vi "Configure Modulation (Amplitude).vi"(0 "VISA resource name":refnum<visa-resource-name>, 1 "Enable AM (T:Enable)":bool=TRUE, 2 "AM Path (1)":u16(ring)=1 items=["1"=1, "2"=2, "Wideband"=3], 5 "AM Mode (1: Normal)":u16(ring)=1 items=["Deep", "Normal"], 7 "AM Type (0: Linear)":u16(ring) items=["Linear", "Exponential"], 9 "Enable Depth Coupling (T:Enable)":bool=TRUE, 11 "error in (no error)":errorcluster, 12 "AM Depth (10 percent)":dbl=10.0, 13 "Wideband AM Sensitivity (20 dB)":dbl=20.0) -> (4 "VISA resource name out":refnum<visa-resource-name>, 15 "error out":errorcluster)   [LabVIEW 2018, in "Agilent PSG MXG Series.lvlib"]
doc: "Configures amplitude modulation.\n\n<B>Notes:</B>\n(1) This VI is <B>NOT</B> valid in E8247C.\n\n(2) For E8257D, E8267D, N5161A, N5162A, N5181A, N5182A, N5183A, this VI is valid only when the instument installs <B>Option UNT</B> (AM, FM, phase modulation).\n\n(3) For N5171B, N5172B, N5181B, N5182B, N5173B, N5183B, this VI is valid only when the instument installs <B>Option UNT</B> (AM, FM, phase modulation)."
uses:
  Agilent PSG MXG Series.lvlib
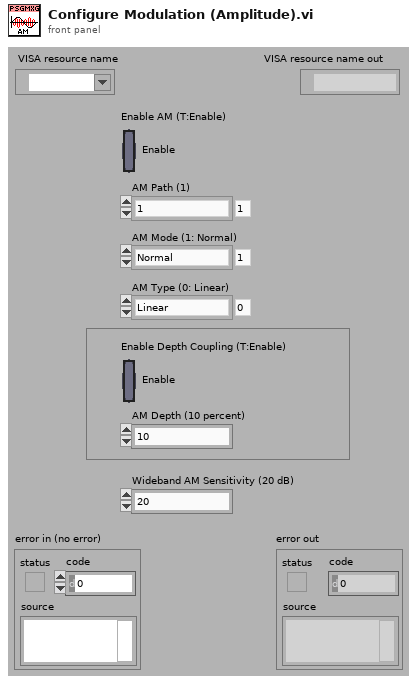
[diagram p1: front panel]
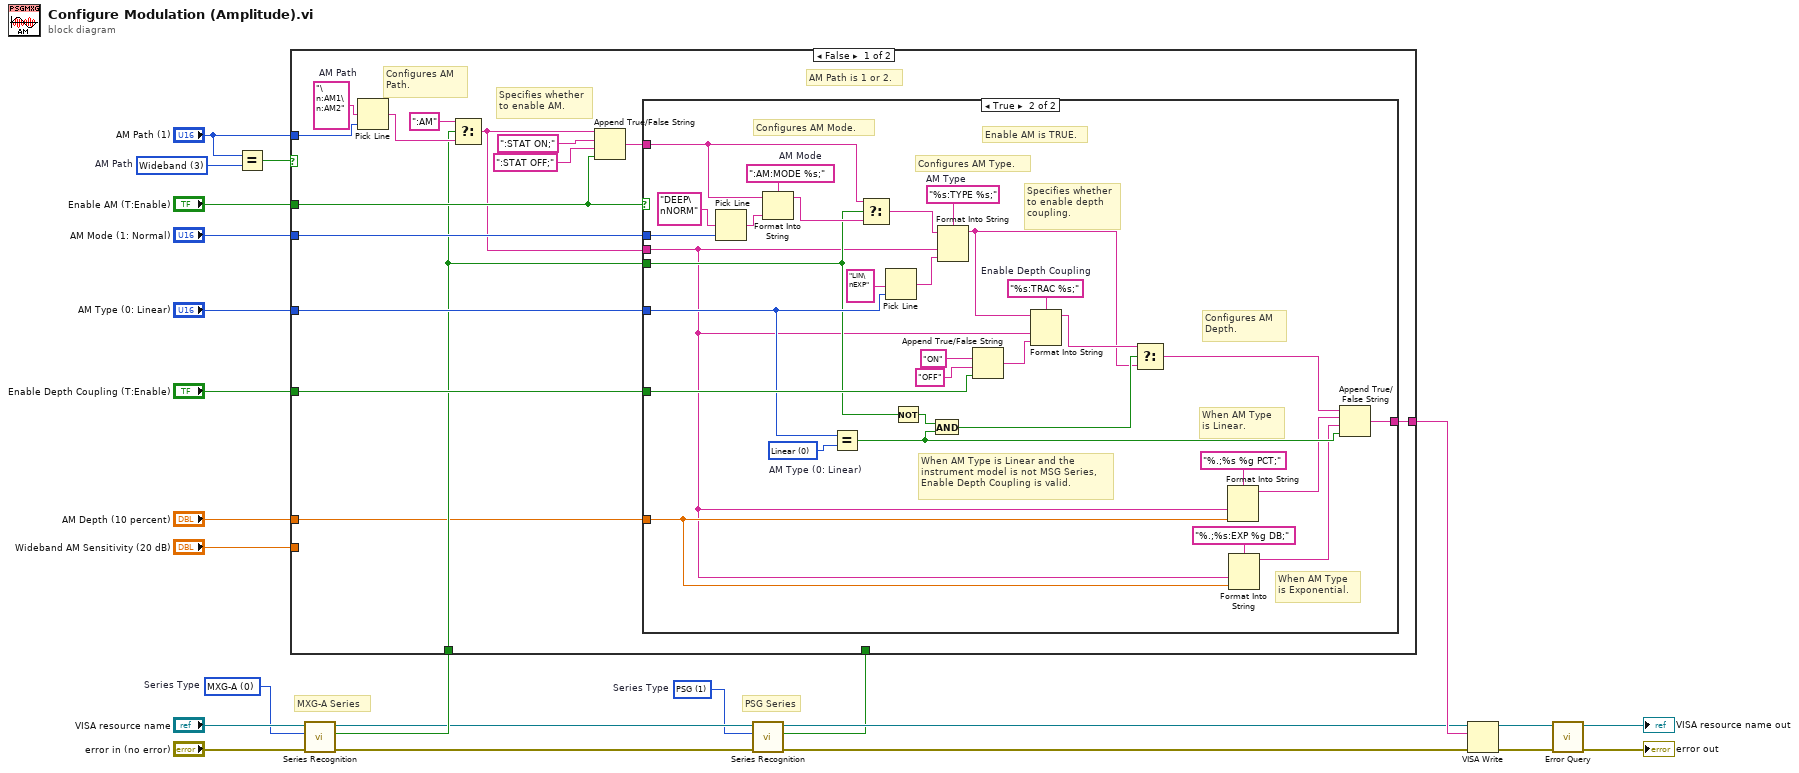
[diagram p0: block diagram]
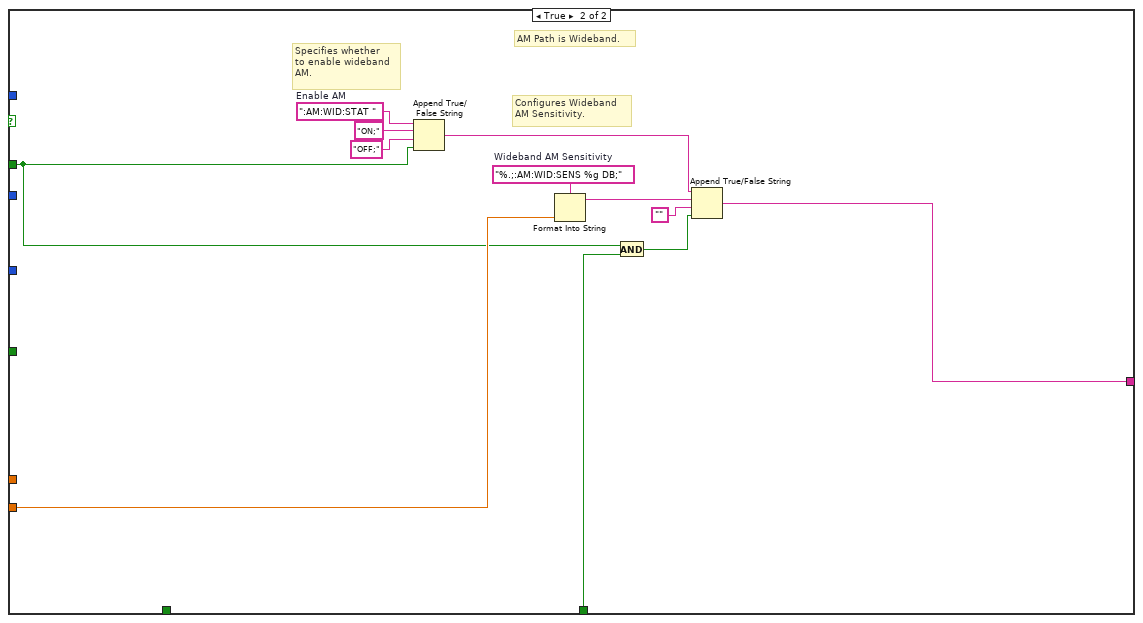
[diagram p3: hidden frame]
diagram:
  w5 = u16 1 items=["MXG-A", "PSG", "PSG-A", "PSG-C", "PSG-D", "MXG-B", "EXG"]  # Series Type
  w8 = u16 0 items=["MXG-A", "PSG", "PSG-A", "PSG-C", "PSG-D", "MXG-B", "EXG"]  # Series Type
  w24 = u16 3 items=["1"=1, "2"=2, "Wideband"=3]  # AM Path
  # "PSG Series"
  # "MXG-A Series"
  n1 = Equal?(x="AM Path (1)", y=w24) -> (x = y?=w23:bool)
  n2 = call "Series Recognition.vi"("error in (no error)"="error in (no error)", "Series Type (0: MXG)"=w8, "VISA resource name"="VISA resource name") -> ("error out"=w6:errorcluster, "Is Series Correct"=w13:bool, "VISA resource name out"=w7:refnum<visa-resource-name>)  [unwired: 6 out]
  n3 = call "Series Recognition.vi"("error in (no error)"=w6, "Series Type (0: MXG)"=w5, "VISA resource name"=w7) -> ("error out"=w2:errorcluster, "Is Series Correct"=w1:bool, "VISA resource name out"=w3:refnum<visa-resource-name>)  [unwired: 6 out]
  n4 = case shown="False" w23 {
    tunnel: "AM Path (1)" -> [w38 _]
    tunnel: "Enable AM (T:Enable)" -> [w32 w76]
    tunnel: "AM Mode (1: Normal)" -> [w35 _]
    tunnel: w13 -> [w29 _]
    tunnel: "AM Type (0: Linear)" -> [w31 _]
    tunnel: "Enable Depth Coupling (T:Enable)" -> [w30 _]
    tunnel: "AM Depth (10 percent)" -> [w27 _]
    tunnel: [w26 w72] -> w4
    tunnel: "Wideband AM Sensitivity (20 dB)" -> [_ w79]
    tunnel: w1 -> [_ w77]
    frame False {
      w39 = "\n:AM1\n:AM2"  # AM Path
      # "Specifies whether\nto enable AM."
      # "Configures AM\nPath."
      # "AM Path is 1 or 2."
      n5 = Pick Line(multi-line string=w39, line index=w38) -> (output string=w34:string)  [unwired: 1 out]
      n6 = Select(t=":AM", s=w29, f=w34) -> (s? t:f=w28:string)
      n7 = Append True/False String(1:w32, 2:":STAT OFF;" ("false string"), 3:":STAT ON;" ("true string"), 4:w28) -> (0:w36:string)
      n8 = case shown="True" w32 {
        tunnel: w36 -> [w40 w67]
        tunnel: w35 -> [_ w68]
        tunnel: w29 -> [_ w53]
        tunnel: w31 -> [_ w56]
        tunnel: w28 -> [_ w41]
        tunnel: w30 -> [_ w57]
        tunnel: w27 -> [_ w47]
        tunnel: [w40 w42] -> w26
        frame False {
          # "Enable AM is FALSE."
        }
        frame True {
          w55 = u16 0 items=["Linear", "Exponential"]  # AM Type (0: Linear)
          w61 = "%s:TRAC %s;"  # Enable Depth Coupling
          w64 = "%s:TYPE %s;"  # AM Type
          w71 = ":AM:MODE %s;"  # AM Mode
          # "When AM Type\nis Exponential."
          # "When AM Type\nis Linear."
          # "Configures AM\nDepth."
          # "When AM Type is Linear and the\ninstrument model is not MSG Series,\nEnable Depth Coupling is valid."
          # "Specifies whether\nto enable depth\ncoupling."
          # "Configures AM Type."
          # "Configures AM Mode."
          # "Enable AM is TRUE."
          n9 = Pick Line(multi-line string="DEEP\nNORM", line index=w68) -> (output string=w70:string)  [unwired: 1 out]
          n10 = Format Into String(format string=w71, initial string=w67, w70) -> (resulting string=w66:string)  [unwired: 1 in, 1 out]
          n11 = Equal?(x=w56, y=w55) -> (x = y?=w46:bool)
          n12 = Select(t=w67, s=w53, f=w66) -> (s? t:f=w65:string)
          n13 = Pick Line(multi-line string="LIN\nEXP", line index=w56) -> (output string=w62:string)  [unwired: 1 out]
          n14 = Not(x=w53) -> (.not. x?=w54:bool)
          n15 = And(x=w54, y=w46) -> (x .and. y?=w52:bool)
          n16 = Format Into String(format string=w64, initial string=w65, w41, w62) -> (resulting string=w50:string)  [unwired: 1 in, 1 out]
          n17 = Append True/False String(1:w57, 2:"OFF" ("false string"), 3:"ON" ("true string")) -> (0:w60:string)  [unwired: 1 out]
          n18 = Format Into String(format string=w61, initial string=w50, w41, w60) -> (resulting string=w51:string)  [unwired: 1 in, 1 out]
          n19 = Select(t=w51, s=w52, f=w50) -> (s? t:f=w43:string)
          n20 = Format Into String(format string="%.;%s %g PCT;", w41, w47) -> (resulting string=w45:string)  [unwired: 2 in, 1 out]
          n21 = Format Into String(format string="%.;%s:EXP %g DB;", w41, w47) -> (resulting string=w44:string)  [unwired: 2 in, 1 out]
          n22 = Append True/False String(1:w46, 2:w44, 3:w45, 4:w43) -> (0:w42:string)
        }
      }
    }
    frame True {
      w80 = "%.;:AM:WID:SENS %g DB;"  # Wideband AM Sensitivity
      w83 = ":AM:WID:STAT "  # Enable AM
      # "Configures Wideband\nAM Sensitivity."
      # "Specifies whether\nto enable wideband\nAM."
      # "AM Path is Wideband."
      n23 = Append True/False String(1:w76, 2:"OFF;" ("false string"), 3:"ON;" ("true string"), 4:w83) -> (0:w78:string)
      n24 = Format Into String(format string=w80, w79) -> (resulting string=w74:string)  [unwired: 2 in, 1 out]
      n25 = And(x=w76, y=w77) -> (x .and. y?=w75:bool)
      n26 = Append True/False String(1:w75, 2:"", 3:w74, 4:w78) -> (0:w72:string)
    }
  }
  n27 = VISA Write(VISA resource name=w3, write buffer=w4, error in (no error)=w2) -> (VISA resource name out=w16:refnum<visa-resource-name>, error out=w15:errorcluster)  [unwired: 1 out]
  n28 = call "Error Query.vi"("error in (no error)"=w15, "VISA resource name"=w16) -> ("error out"=→"error out":errorcluster, "VISA resource name out"=→"VISA resource name out":refnum<visa-resource-name>)  [unwired: 8 out]
